vi "Create (String).vi"(10 "error in (no error)":errorcluster, 11 "URI String":string) -> (2 "error out":errorcluster, 3 "URI out":refnum<class "URI.lvclass">)   [LabVIEW 2020, in "URI.lvlib" / "URI.lvclass"]
uses:
  URI.lvclass
  URI.lvclass/URI.ctl
  URI.lvlib
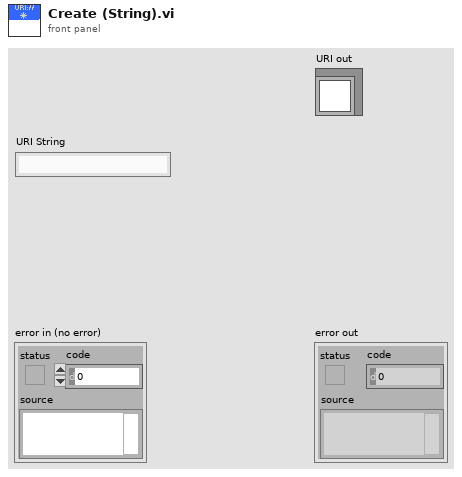
[diagram p1: front panel]
types:
  T1 = typedef "URI.lvlib/URI Components.ctl" = cluster{"Scheme":string, "User Info":string, "Host":string, "Port":string, "Path":string, "Query":string, "Fragment":string}
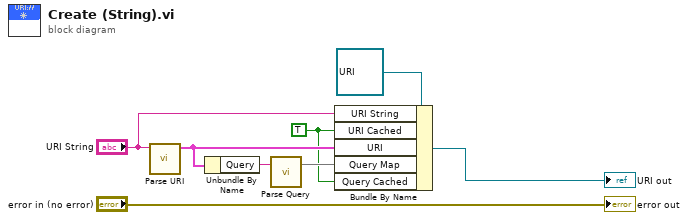
[diagram p0: block diagram]
diagram:
  w1 = TRUE ("String Cached")
  n1 = call "Parse URI.vi"("URI String"="URI String") -> ("Parsed Components"=w4:T1)  [unwired: 9 in, 1 out]
  n2 = Unbundle By Name(w4) -> ("Query"=w3:string)
  n3 = call "Parse Query.vi"("Query String"=w3) -> ("Query Map"=w2:map{string, string})  [unwired: 6 in]
  n4 = Bundle By Name(cluster=refnum<class "URI.lvclass"> refnum ("URI in"), "URI String"="URI String", "URI Cached"=w1, "URI"=w4, "Query Map"=w2, "Query Cached"=w1) -> (→"URI out":refnum<class "URI.lvclass">)
  "error out" <- "error in (no error)"
